vi "ExSubCenterStrip.vi"(2 "error in (no error)":errorcluster, 3 "Camera Handle":u32) -> (0 "error out":errorcluster, 1 "Camera Handle":u32)   [LabVIEW 2010]
uses:
  GlobalExposure.vi
  GlobalFramesToStr.vi
  GlobalAcquireFocusFlag.vi
  GlobalCCDMaxDim.vi
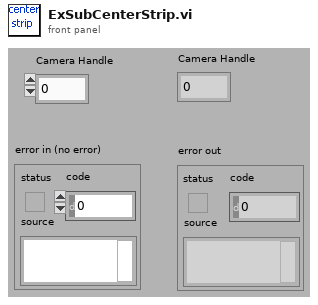
[diagram p1: front panel]
types:
  T1 = cluster{i32, "CCD Max X":u32, i32, i32, i32, i32}
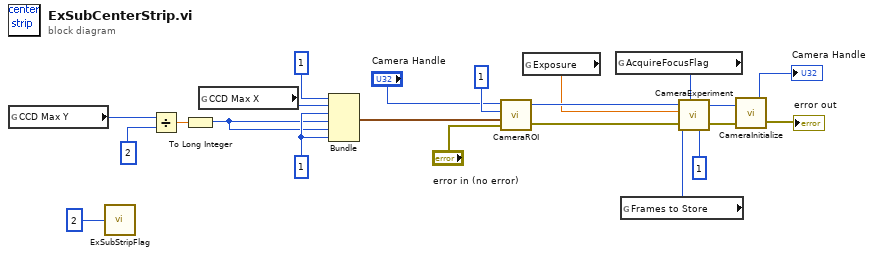
[diagram p0: block diagram]
diagram:
  w11 = 1
  n1 = global read "GlobalCCDMaxDim.vi" "CCD Max Y"() -> (w7:u32)
  n2 = call "ExSubStripFlag.vi"("Binning \nUser = 1\nCenter = 2\nFull = 3"=2) -> ()
  n3 = Divide(x=w7, y=2) -> (x/y=w6:dbl)
  n4 = To Long Integer(number=w6) -> (32bit integer=w5:i32)
  n5 = global read "GlobalCCDMaxDim.vi" "CCD Max X"() -> (w14:u32)
  n6 = Bundle(1, "CCD Max X"=w14, w11, w5, w5, w11) -> (w13:T1)  [unwired: 1 in]
  n7 = call <userlib>:"CameraROI.vi"("error in"="error in (no error)", "ROI Params"=w13, "ROI Index"=1, "Camera Handle"="Camera Handle") -> ("error out"=w20:errorcluster, "Camera Handle"=w22:u32)
  n8 = global read "GlobalExposure.vi" "Exposure"() -> (w17:dbl)
  n9 = global read "GlobalAcquireFocusFlag.vi" "AcquireFocusFlag"() -> (w15:u32)
  n10 = global read "GlobalFramesToStr.vi" "Frames to Store"() -> (w16:u32)
  n11 = call <userlib>:"CameraExperiment.vi"("Number of Accumulations"=1, "Acquire / Focus Flag"=w15, "error in"=w20, "Number of Images"=w16, "Exposure (sec)"=w17, "Camera Handle"=w22) -> ("error out"=w19:errorcluster, "Camera Handle"=w21:u32)
  n12 = call <userlib>:"CameraInitialize.vi"("error in"=w19, "Camera Handle"=w21) -> ("error out"=→"error out":errorcluster, "Camera Handle"=→"Camera Handle":u32)
